vi "Main.vi"(11 "Module Admin":refnum<class "Delacor_lib_QMH_Cloneable Module Admin.lvclass">) -> ()   [LabVIEW 2024, in "RaspberryPiPico.lvlib"]
doc: "This template is based off of the Queued Message Handler design pattern and the Queued Message Handler project template that ships with LabVIEW.\n\nThe main difference is that the queue is private to this module and communication between modules is performed via Broadcast and Request events.\n\nRequest events are wrapped in public API methods and are handled in the Event Handling Loop (EHL) of this VI. Any module can register for Broadcast events sent by this module. The EHL generates messages based on user interface actions.\n\nThe Message Handling Loop (MHL) processes messages generated by the EHL, or by other messages. The messages are string values, so new messages can be added easily to the Message Cases case structure in the MHL. Each message cluster can also provide an optional value for Message Data, which is a variant that can be converted to whatever message-specific data is required.\n_____\nBased on DQMH Dev Tools: Project Template 7.1.0.1503."
uses:
  RaspberryPiPico.lvlib
  <vilib>/Delacor/Delacor QMH/Libraries/Cloneable Module Admin_class/Delacor_lib_QMH_Cloneable Module Admin.lvclass
  C:/Program Files (x86)/National Instruments/LabVIEW 2024/vi.lib/Delacor/Delacor QMH/Libraries/Module Admin_class/Delacor_lib_QMH_Module Admin.lvclass
  Module Data--cluster.ctl
  <vilib>/Delacor/Delacor QMH/Libraries/Cloneable Module Admin_class/Delacor_lib_QMH_Cloneable Module Admin.lvclass/Delacor_lib_QMH_Cloneable Module Admin.ctl
  <vilib>/Delacor/Delacor QMH/Libraries/Message Queue_class/Delacor_lib_QMH_Message Queue.lvclass/Delacor_lib_QMH_Message Queue.ctl
  Stop Argument--cluster.ctl
  <vilib>/Delacor/Delacor QMH/Libraries/Module Admin_class/Delacor_lib_QMH_Module Admin.lvclass/Delacor_lib_QMH_Module Admin.ctl
  Initialize Instrument Argument--cluster.ctl
  Initialize Instrument (Reply Payload)--cluster.ctl
  <instrlib>/HandsOnPi2040/cti-drivers-lv-visa-main/CTI-Visa/Identity.ctl
  <vilib>/Utility/miscctls.llb/LVPointTypeDef.ctl
  <vilib>/Delacor/Delacor QMH/Libraries/Cloneable Module Admin_class/Delacor_lib_QMH_Get Module ID.vi
  <vilib>/Delacor/Delacor QMH/Libraries/Message Queue_class/Delacor_lib_QMH_Enqueue Message (Single).vi
  <vilib>/Delacor/Delacor QMH/Libraries/Module Admin_class/Delacor_lib_QMH_Get External Launch.vi
  <vilib>/Delacor/Delacor QMH/Libraries/Message Queue_class/Delacor_lib_QMH_Message Queue.lvclass
  <instrlib>/HandsOnPi2040/cti-drivers-lv-visa-main/CTI-Visa/CTI-Visa.lvlib
  <instrlib>/HandsOnPi2040/HandsOnPi2040.lvlib
panel:
  out "error out":errorcluster
  out "Status":string
  in  "Simulate EHL Error":bool
  in  "Simulate MHL Error":bool
  # "Other processes communicate with this Module via its Public API (wrappers for its Request Events).\n\nThis Module communicates with other processes via its Broadcast Events.\nAny process that wants to receive these messages can register for this module's Broadcast events."
  # "This template is for the DQMH framework. See the block diagram for more information on how to use this template."
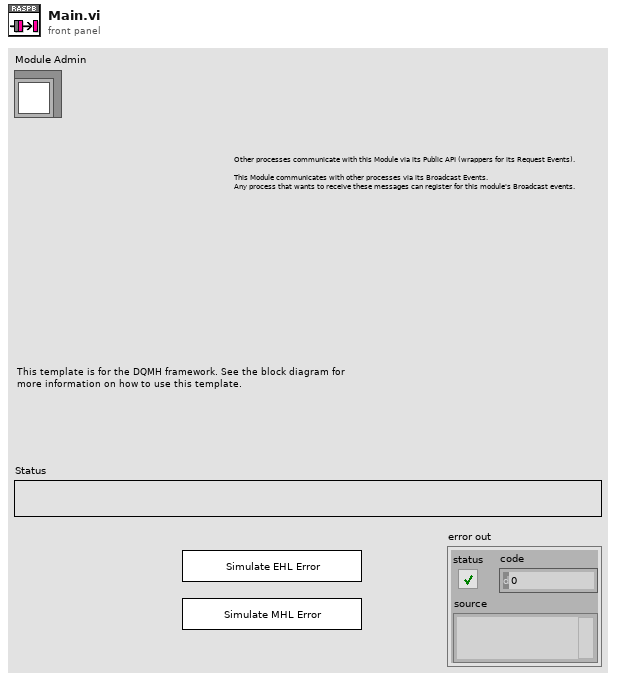
[diagram p1: front panel]
types:
  T1 = typedef "RaspberryPiPico.lvlib/Request Events--cluster.ctl" = cluster{"Stop Module":refnum<user-event>, "Show Panel":refnum<user-event>, "Hide Panel":refnum<user-event>, "Show Diagram":refnum<user-event>, "Get Module Execution Status":refnum<user-event>, "Initialize Instrument":refnum<user-event>, "Local Instance":T2}
  T2 = typedef "RaspberryPiPico.lvlib/Local Instance Request Events--cluster.ctl" = cluster{"Start Continuous Acquisition":refnum<user-event>}
  T3 = typedef "RaspberryPiPico.lvlib/Module Data--cluster.ctl" = cluster{"Status":string, "VISA resource name":refnum<visa-resource-name>}
  T4 = enum32{"invalid lock state", "Not Locked", "Locked (No Password)", "Password-protected"}
  T5 = typedef "RaspberryPiPico.lvlib/Stop Argument--cluster.ctl" = cluster{"Module ID":i32, "Origin":string, "Exit via Stop Module Req?":bool, "Wait for Module to stop?":bool}
  T6 = typedef "RaspberryPiPico.lvlib/Initialize Instrument Argument--cluster.ctl" = cluster{"Module ID":i32, "VISA resource name":refnum<visa-resource-name>, "Wait Notifier":refnum<notifier>, "wait for reply":bool}
  T7 = typedef "LVPointTypeDef.ctl" = cluster{"Horizontal":i16, "Vertical":i16}
  T8 = enum32{"Invalid", "Standard", "Closed", "Hidden", "Minimized", "Maximized"}
  T9 = typedef "RaspberryPiPico.lvlib/Initialize Instrument (Reply Payload)--cluster.ctl" = cluster{"Module ID":i32, "Identity":T10, "error":errorcluster}
  T10 = typedef "CTI-Visa.lvlib/Identity.ctl" = cluster{"Vendor":string, "Model":string, "Serial":string, "Version":string}
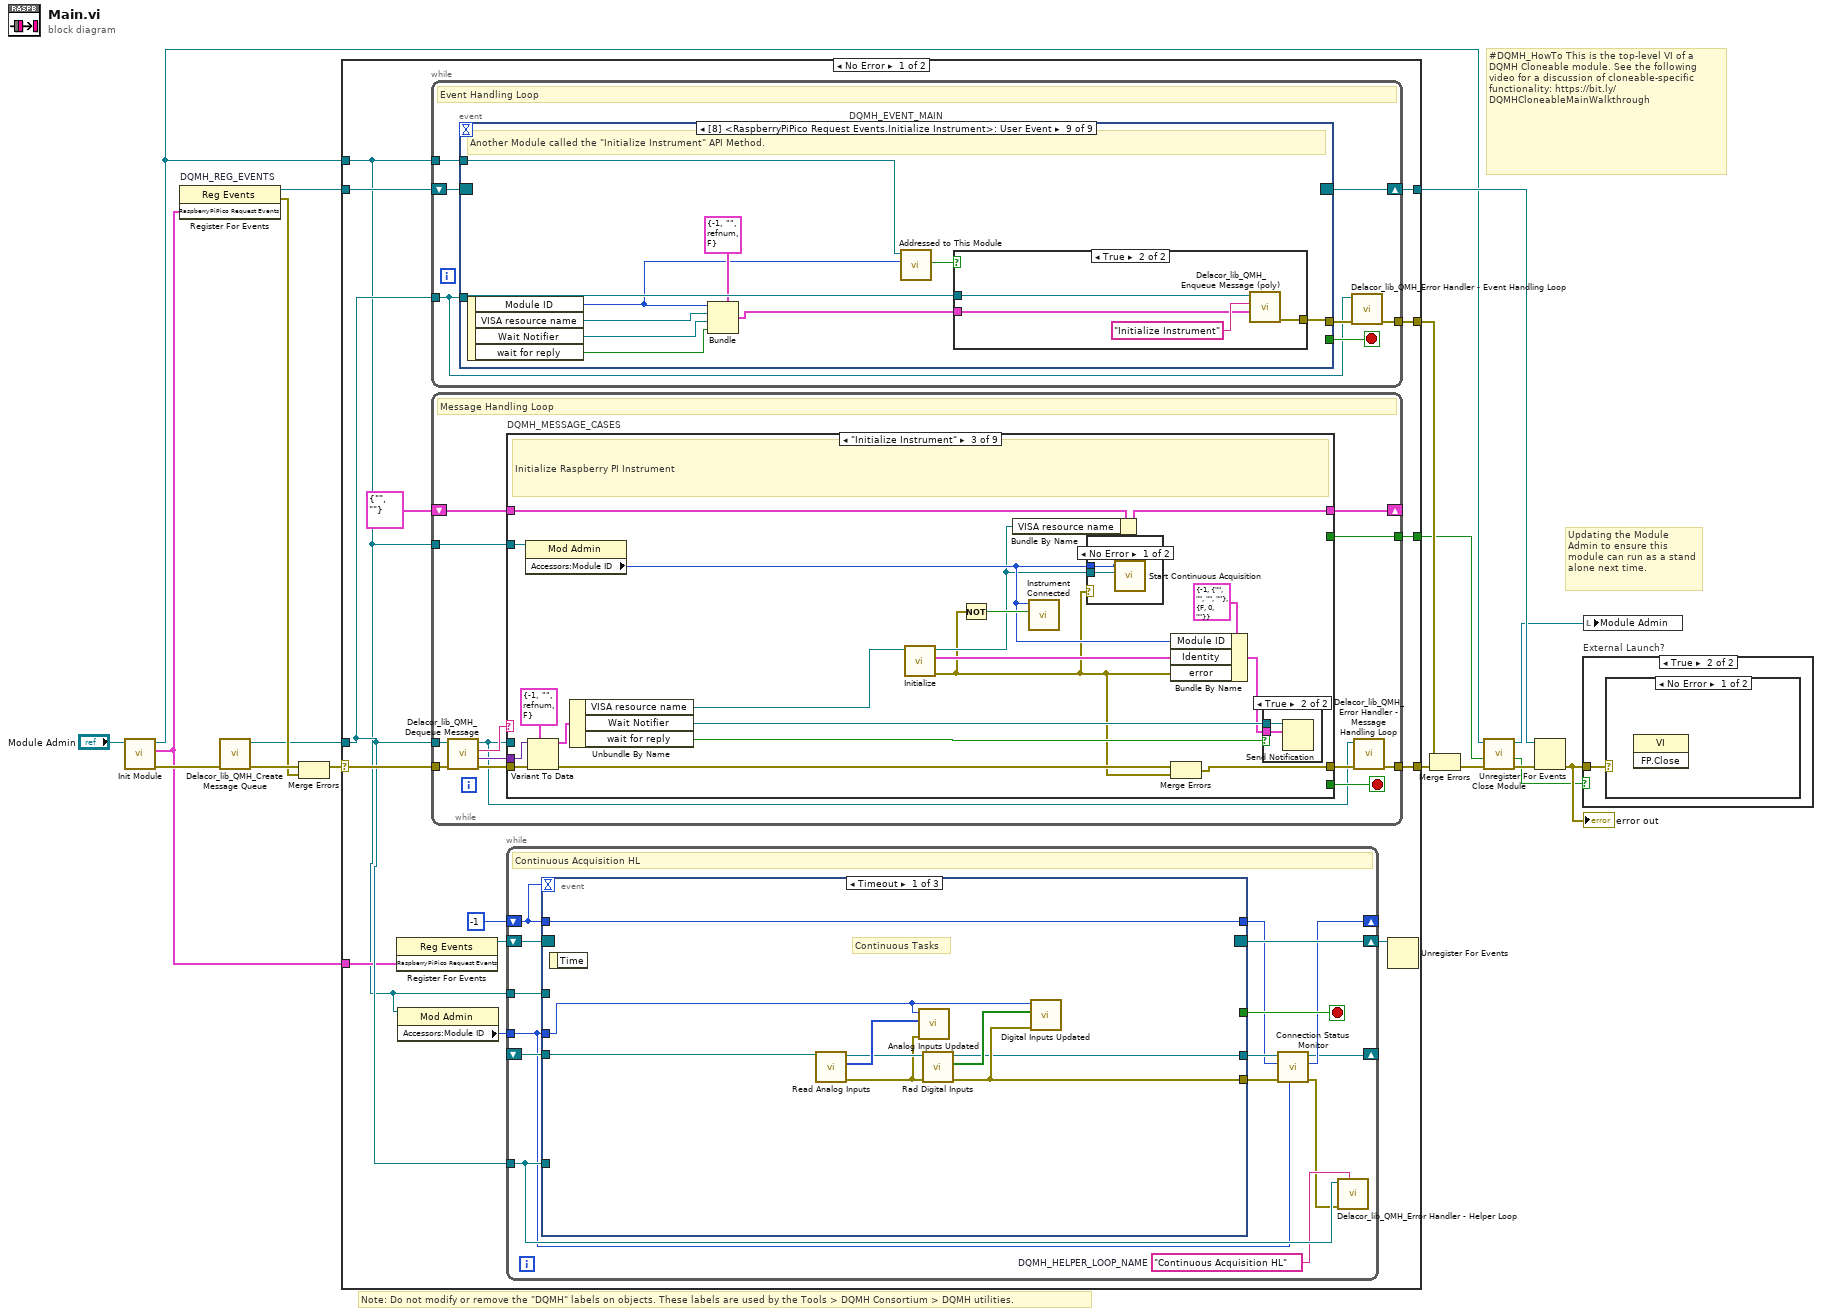
[diagram p0: block diagram]
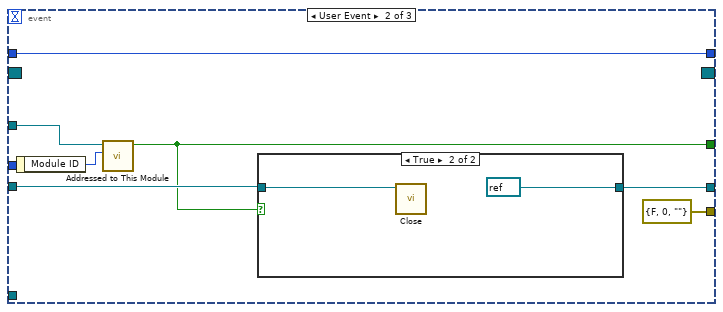
[diagram p2: hidden frame]
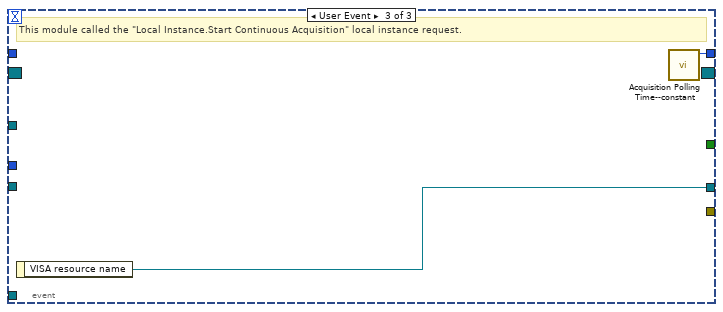
[diagram p4: hidden frame]
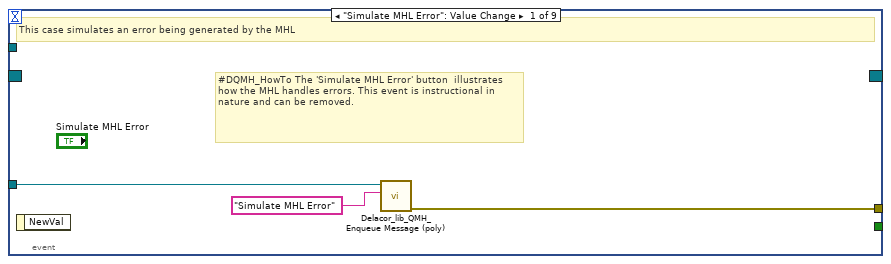
[diagram p5: hidden frame]
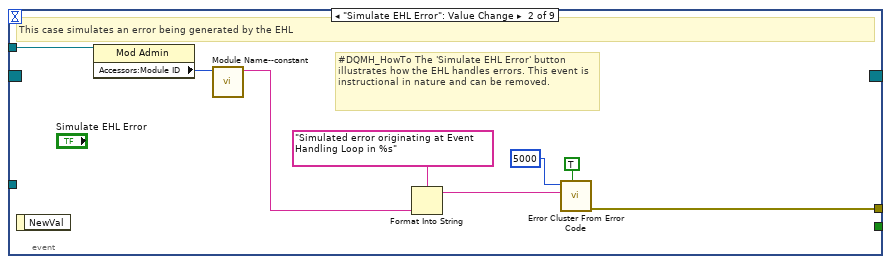
[diagram p6: hidden frame]
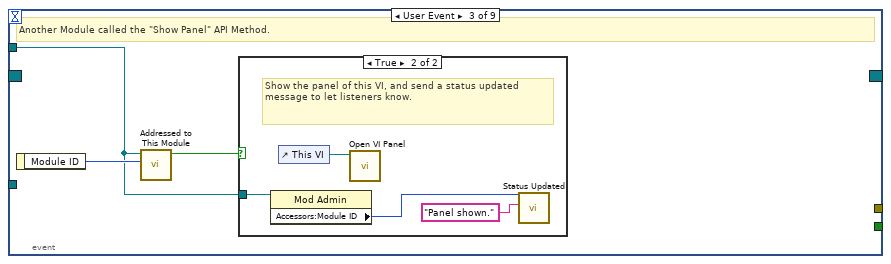
[diagram p7: hidden frame]
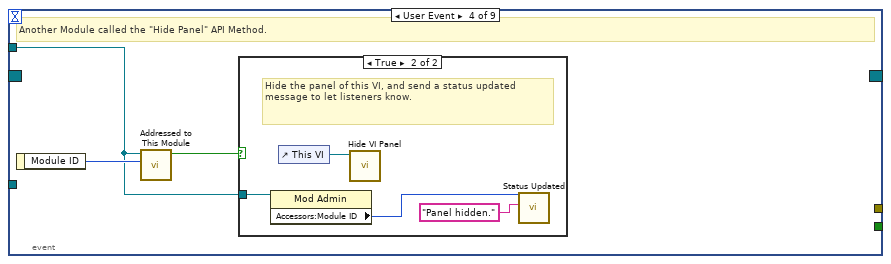
[diagram p9: hidden frame]
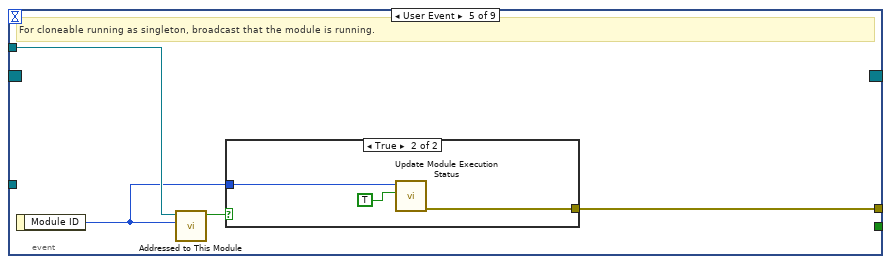
[diagram p11: hidden frame]
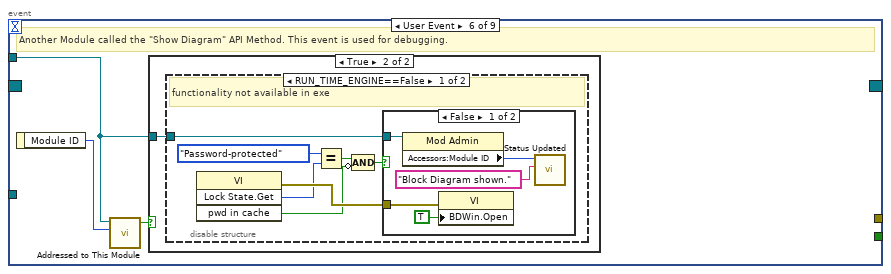
[diagram p13: hidden frame]
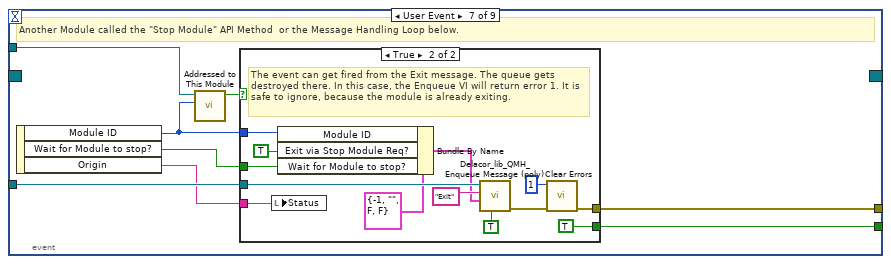
[diagram p17: hidden frame]
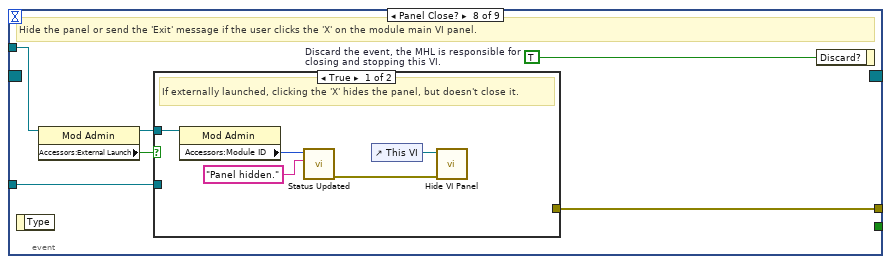
[diagram p19: hidden frame]
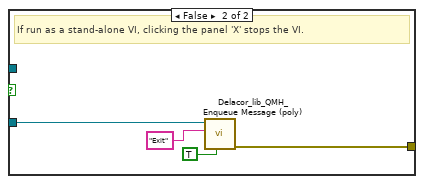
[diagram p20: hidden frame]
diagram:
  # "#DQMH_HowTo This is the top-level VI of a DQMH Cloneable module. See the following video for a discussion of cloneable-specific functionality: https://bit.ly/DQMHCloneableMainWalkthrough"
  # "Note: Do not modify or remove the \"DQMH\" labels on objects. These labels are used by the Tools > DQMH Consortium > DQMH utilities."
  # "Updating the Module Admin to ensure this module can run as a stand alone next time."
  n1 = call "Init Module.vi"("Cloneable Module Admin in"="Module Admin") -> ("error out"=w15:errorcluster, "RaspberryPiPico Request Events"=w1:T1, "Cloneable Module Admin out"=w5:refnum<class "Delacor_lib_QMH_Cloneable Module Admin.lvclass">)  [unwired: 8 in]
  n2 = register-events "DQMH_REG_EVENTS"(w1) -> (reference out=w8:refnum<event-registration>, error out=w10:errorcluster)  [unwired: 2 in]
  n3 = call <vilib>:"Delacor_lib_QMH_Create Message Queue.vi"("error in"=w15) -> ("error out"=w12:errorcluster, "Message Queue"=w7:refnum<class "Delacor_lib_QMH_Message Queue.lvclass">)  [unwired: 9 in]
  n4 = Merge Errors(w12, w10) -> (w11:errorcluster)
  n5 = case shown="No Error" w11 {
    selector: w11 -> [w30 w307]
    tunnel: [w32 w306] -> w16
    tunnel: [w29 w305] -> w9
    tunnel: w8 -> [w27 w305]
    tunnel: w7 -> [w26 w298]
    tunnel: [w31 _] -> w17
    tunnel: w5 -> [w20 w301]
    tunnel: [w25 _] -> w3
    tunnel: w1 -> [w24 _]
    frame No Error {
      n6 = register-events ("DQMH_HELPER_REGFOREVENTS")(w24) -> (reference out=w22:refnum<event-registration>)  [unwired: 2 in, 1 out]
      n7 = property class="Mod Admin"(reference=w20) -> ("Accessors:Module ID"=w19:i32)  [unwired: 1 in, 2 out]
      n8 = while {
        tunnel: w26 -> [w70]
        shift-right: [w73] -> w29
        shift-left: w27 -> [w74]
        tunnel: [w75] -> w31
        tunnel: w20 -> [w71]
        stop <- w72 stop-if-true
        # "Event Handling Loop"
        n9 = event "DQMH_EVENT_MAIN" shown="[8] <RaspberryPiPico Request Events.Initialize Instrument>: User Event" {
          selector: w74 -> [_ _ _ _ _ _ _ _ _]
          dyn-events: [_ _ _ _ _ _ _ _ _] -> w73
          timeout: _ -> [_ _ _ _ _ _ _ _ _]
          tunnel: [_ _ _ _ _ _ w128 _ _] -> w72
          tunnel: w70 -> [w78 _ _ _ _ _ w131 w148 w169]
          tunnel: [w79 w87 _ _ w105 _ w132 w151 w170] -> w76
          tunnel: w71 -> [_ w86 w88 w95 w103 w109 w130 w149 w167]
          event "Simulate MHL Error": Value Change {
            # "#DQMH_HowTo The 'Simulate MHL Error' button  illustrates how the MHL handles errors. This event is instructional in nature and can be removed."
            # "This case simulates an error being generated by the MHL"
            n10 = event-data() -> ()  [unwired: 1 in, 1 out]
            n11 = call-poly <vilib>:"Delacor_lib_QMH_Enqueue Message (poly).vi"("Message"="Simulate MHL Error", "Message Queue in"=w78) -> ("error out"=w79:errorcluster)  [unwired: 8 in, 1 out]
          }
          event "Simulate EHL Error": Value Change {
            # "#DQMH_HowTo The 'Simulate EHL Error' button  illustrates how the EHL handles errors. This event is instructional in nature and can be removed."
            # "This case simulates an error being generated by the EHL"
            n12 = event-data() -> ()  [unwired: 1 in, 1 out]
            n13 = property on="Property Node" class="Mod Admin"(reference=w86) -> ("Accessors:Module ID"=w85:i32)  [unwired: 1 in, 2 out]
            n14 = call "Module Name--constant.vi"("Module ID"=w85) -> ("Module Name"=w80:string)  [unwired: 10 in]
            n15 = Format Into String(format string="Simulated error originating at Event Handling Loop in %s", w80) -> (resulting string=w83:string)  [unwired: 2 in, 1 out]
            n16 = call <vilib>:"Error Cluster From Error Code.vi"("show call chain? (False)"=TRUE, "error message (\"\")"=w83, "error code (0)"=5000) -> ("error out"=w87:errorcluster)  [unwired: 6 in]
          }
          event User Event {
            # "Another Module called the \"Show Panel\" API Method."
            n17 = event-data() -> ("Module ID"=w89:i32)  [unwired: 1 in]
            n18 = call "Addressed to This Module.vi"("Module ID from Argument"=w89, "Module Admin"=w88) -> ("Addressed to this instance?"=w90:bool)  [unwired: 8 in, 1 out]
            n19 = case shown="True" w90 {
              tunnel: w88 -> [_ w92]
              frame False {
              }
              frame True {
                # "Show the panel of this VI, and send a status updated message to let listeners know."
                n20 = property on="Property Node" class="Mod Admin"(reference=w92) -> ("Accessors:Module ID"=w91:i32)  [unwired: 1 in, 2 out]
                n21 = control-ref of="This VI"() -> (w94:refnum<vi>)
                n22 = call "Open VI Panel.vi"("VI"=w94) -> ()  [unwired: 10 in, 1 out]
                n23 = call "Status Updated.vi"("Status"="Panel shown." ("format string"), "Module ID"=w91) -> ()  [unwired: 9 in, 1 out]
              }
            }
          }
          event User Event {
            # "Another Module called the \"Hide Panel\" API Method."
            n24 = event-data() -> ("Module ID"=w96:i32)  [unwired: 1 in]
            n25 = call "Addressed to This Module.vi"("Module ID from Argument"=w96, "Module Admin"=w95) -> ("Addressed to this instance?"=w97:bool)  [unwired: 8 in, 1 out]
            n26 = case shown="True" w97 {
              tunnel: w95 -> [_ w99]
              frame False {
              }
              frame True {
                # "Hide the panel of this VI, and send a status updated message to let listeners know."
                n27 = property on="Property Node" class="Mod Admin"(reference=w99) -> ("Accessors:Module ID"=w98:i32)  [unwired: 1 in, 2 out]
                n28 = control-ref of="This VI"() -> (w101:refnum<vi>)
                n29 = call "Hide VI Panel.vi"("VI"=w101) -> ()  [unwired: 10 in, 1 out]
                n30 = call "Status Updated.vi"("Status"="Panel hidden." ("format string"), "Module ID"=w98) -> ()  [unwired: 9 in, 1 out]
              }
            }
          }
          event User Event {
            # "For cloneable running as singleton, broadcast that the module is running."
            n31 = event-data() -> ("Module ID"=w102:i32)  [unwired: 1 in]
            n32 = call "Addressed to This Module.vi"("Module ID from Argument"=w102, "Module Admin"=w103) -> ("Addressed to this instance?"=w104:bool)  [unwired: 8 in, 1 out]
            n33 = case shown="True" w104 {
              tunnel: [_ w108] -> w105
              tunnel: w102 -> [_ w107]
              frame False {
              }
              frame True {
                n34 = call "Update Module Execution Status.vi"("Running?"=TRUE, "Module ID"=w107) -> ("error out"=w108:errorcluster)  [unwired: 9 in]
              }
            }
          }
          event User Event {
            # "Another Module called the \"Show Diagram\" API Method. This event is used for debugging."
            n35 = event-data() -> ("Module ID"=w110:i32)  [unwired: 1 in]
            n36 = call "Addressed to This Module.vi"("Module ID from Argument"=w110, "Module Admin"=w109) -> ("Addressed to this instance?"=w111:bool)  [unwired: 8 in, 1 out]
            n37 = case shown="True" w111 {
              tunnel: w109 -> [_ w112]
              frame False {
              }
              frame True {
                n38 = disable-structure shown="RUN_TIME_ENGINE==False" {
                  disable-tunnel: w112 -> [w113 _]
                  frame condition #0 (active) {
                    # "functionality not available in exe"
                    n39 = invoke on="Invoke Node" class="VI" method="Lock State.Get"() -> (error out=w119:errorcluster, "Get Lock State"=w118:T4, "pwd in cache"=w115:bool)  [unwired: 4 in, 1 out]
                    n40 = Equal?(x=T4."Password-protected", y=w118) -> (x = y?=w116:bool)
                    n41 = Compound Arithmetic op=AND(w116, invert w115) -> (w114:bool)
                    n42 = case shown="False" w114 {
                      tunnel: w119 -> [w124 _]
                      tunnel: w113 -> [w121 _]
                      frame False {
                        n43 = property on="Property Node" class="Mod Admin"(reference=w121) -> ("Accessors:Module ID"=w120:i32)  [unwired: 1 in, 2 out]
                        n44 = property on="Property Node" class="VI"(error in=w124, "BDWin.Open"=TRUE ("Block Diagram Window:Open")) -> ()  [unwired: 1 in, 2 out]
                        n45 = call "Status Updated.vi"("Status"="Block Diagram shown." ("format string"), "Module ID"=w120) -> ()  [unwired: 9 in, 1 out]
                      }
                      frame True {
                        # "Password-protected VI, and the password is not in the cache. Do not show the diagram."
                      }
                    }
                  }
                  frame condition #1 {
                  }
                }
              }
            }
          }
          event User Event {
            # "Another Module called the \"Stop Module\" API Method  or the Message Handling Loop below."
            n46 = event-data() -> ("Module ID"=w126:i32, "Wait for Module to stop?"=w127:bool, "Origin"=w125:string)  [unwired: 1 in]
            n47 = call "Addressed to This Module.vi"("Module ID from Argument"=w126, "Module Admin"=w130) -> ("Addressed to this instance?"=w129:bool)  [unwired: 8 in, 1 out]
            n48 = case shown="True" w129 {
              tunnel: [_ w144] -> w132
              tunnel: w131 -> [_ w140]
              tunnel: [_ TRUE] -> w128
              tunnel: w127 -> [_ w135]
              tunnel: w126 -> [_ w137]
              tunnel: w125 -> [_ w133]
              frame False {
              }
              frame True {
                # "The event can get fired from the Exit message. The queue gets destroyed there. In this case, the Enqueue VI will return error 1. It is safe to ignore, because the module is already exiting."
                n49 = local write "Status"(w133) -> ()
                n50 = Bundle By Name(cluster=T5 {"Module ID"=-1, "Origin"="", "Exit via Stop Module Req?"=FALSE, "Wait for Module to stop?"=FALSE} ("Stop Argument"), "Module ID"=w137, "Exit via Stop Module Req?"=TRUE, "Wait for Module to stop?"=w135) -> (w134:T5)
                n51 = call-poly <vilib>:"Delacor_lib_QMH_Enqueue Message (poly).vi"("Priority Message? (F)"=TRUE, "Message Data"=w134, "Message"="Exit", "Message Queue in"=w140) -> ("error out"=w145:errorcluster)  [unwired: 6 in, 1 out]
                n52 = call <vilib>:"Clear Errors.vi"("error in (no error)"=w145, "specific error code to clear (0: all)"=1) -> ("error out"=w144:errorcluster)  [unwired: 4 in, 1 out]
              }
            }
          }
          event Panel Close? {
            w150 = TRUE  # Discard the event, the MHL is responsible for closing and stopping this VI.
            # "Hide the panel or send the 'Exit' message if the user clicks the 'X' on the module main VI panel."
            n53 = event-data() -> ()  [unwired: 1 in, 1 out]
            n54 = property on="Property Node" class="Mod Admin"(reference=w149) -> (reference out=w146:refnum<class "Delacor_lib_QMH_Cloneable Module Admin.lvclass">, "Accessors:External Launch"=w147:bool)  [unwired: 1 in, 1 out]
            n55 = case shown="True" w147 {
              tunnel: w148 -> [_ w159]
              tunnel: [_ w160] -> w151
              tunnel: w146 -> [w153 _]
              frame True {
                # "If externally launched, clicking the 'X' hides the panel, but doesn't close it."
                n56 = property on="Property Node" class="Mod Admin"(reference=w153) -> ("Accessors:Module ID"=w152:i32)  [unwired: 1 in, 2 out]
                n57 = call "Status Updated.vi"("Status"="Panel hidden." ("format string"), "Module ID"=w152) -> ("error out"=w156:errorcluster)  [unwired: 9 in]
                n58 = control-ref of="This VI"() -> (w155:refnum<vi>)
                n59 = call "Hide VI Panel.vi"("error in"=w156, "VI"=w155) -> ()  [unwired: 9 in, 1 out]
              }
              frame False {
                # "If run as a stand-alone VI, clicking the panel 'X' stops the VI."
                n60 = call-poly <vilib>:"Delacor_lib_QMH_Enqueue Message (poly).vi"("Priority Message? (F)"=TRUE, "Message"="Exit", "Message Queue in"=w159) -> ("error out"=w160:errorcluster)  [unwired: 7 in, 1 out]
              }
            }
            n61 = event-data ("Event Filter Node")("Discard?"=w150) -> ()  [unwired: 1 in, 1 out]
          }
          event User Event {
            # "Another Module called the \"Initialize Instrument\" API Method."
            n62 = event-data() -> ("Module ID"=w164:i32, "VISA resource name"=w163:refnum<visa-resource-name>, "Wait Notifier"=w162:refnum<notifier>, "wait for reply"=w161:bool)  [unwired: 1 in]
            n63 = Bundle(cluster=T6 {"Module ID"=-1, "VISA resource name"="", "Wait Notifier"=refnum, "wait for reply"=FALSE} ("Initialize Instrument Argument"), "Module ID"=w164, "VISA resource name"=w163, "Wait Notifier"=w162, "wait for reply"=w161) -> (w165:T6)
            n64 = call "Addressed to This Module.vi"("Module ID from Argument"=w164, "Module Admin"=w167) -> ("Addressed to this instance?"=w168:bool)  [unwired: 8 in, 1 out]
            n65 = case shown="True" w168 {
              tunnel: w169 -> [_ w173]
              tunnel: w165 -> [_ w171]
              tunnel: [_ w174] -> w170
              frame False {
              }
              frame True {
                n66 = call-poly <vilib>:"Delacor_lib_QMH_Enqueue Message (poly).vi"("Message Data"=w171, "Message"="Initialize Instrument", "Message Queue in"=w173) -> ("error out"=w174:errorcluster)  [unwired: 7 in, 1 out]
              }
            }
          }
        }
        n67 = call-dynamic "Delacor_lib_QMH_Error Handler - Event Handling Loop.vi"("error in"=w76, "Message Queue in"=w70) -> ("dup error in"=w75:errorcluster)  [unwired: 8 in, 1 out]
      }
      n68 = while {
        tunnel: w26 -> [w175]
        shift-right: [w182] -> _
        shift-left: T3 {"Status"="", "VISA resource name"=""} ("Data Cluster") -> [w183]
        tunnel: w30 -> [w186]
        tunnel: [w184] -> w32
        tunnel: w20 -> [w177]
        tunnel: [w176] -> w25
        stop <- w181 stop-if-true
        # "Message Handling Loop"
        n69 = call-dynamic "Delacor_lib_QMH_Dequeue Message.vi"("error in"=w186, "Message Queue in"=w175) -> ("error out"=w185:errorcluster, "Message Data"=w179:variant, "Message"=w180:string, "Message Queue out"=w178:refnum<class "Delacor_lib_QMH_Message Queue.lvclass">)  [unwired: 6 in]
        n70 = case "DQMH_MESSAGE_CASES" shown="\"Initialize Instrument\"" w180 {
          selector: w180 -> [_ _ _ _ _ _ _ _ w287]
          tunnel: w178 -> [_ _ _ _ _ w240 _ w279 _]
          tunnel: w185 -> [w206 w210 w229 w236 w238 w250 w267 w285 w296]
          tunnel: [w204 w210 w227 w235 w238 w246 w266 w280 w297] -> w187
          tunnel: w183 -> [w197 w209 w226 w234 w237 w244 w264 w269 w294]
          tunnel: [w196 w209 w216 w234 w237 w244 w264 w269 w294] -> w182
          tunnel: [_ _ _ _ _ _ _ w278 _] -> w181
          tunnel: w179 -> [_ _ w225 _ _ w243 _ w276 _]
          tunnel: w177 -> [w192 _ w218 _ _ w242 w262 w271 w293]
          tunnel: [_ _ _ _ _ _ _ w274 _] -> w176
          frame "Initialize" {
            w189 = "Initial Message" ("Initial Message")
            # "#DQMH_CodeNeeded - Initialize the appearance of the front panel."
            # "#DQMH_CodeNeeded - Initialize your state data here."
            # "Initialize - Any operation that needs to be done before the module can receive messages. Synchronize Caller Events.vi will inform Start Module.vi that the module has launched and is ready to receive messages. Module Did Init.vi will broadcast that the module initialized."
            n71 = call "Synchronize Caller Events.vi"("error in"=w206, "Module Admin"=w192) -> ("error out"=w205:errorcluster, "Module Admin out"=w191:refnum<class "Delacor_lib_QMH_Cloneable Module Admin.lvclass">)  [unwired: 8 in]
            n72 = property on="Property Node" class="Mod Admin"(reference=w191) -> ("Accessors:Module ID"=w188:i32, "Accessors:External Launch"=w193:bool)  [unwired: 1 in, 2 out]
            n73 = call "Module Name--constant.vi"("Module ID"=w188) -> ("Module Name"=w201:string)  [unwired: 10 in]
            n74 = property on="Property Node" class="VI"("Front Panel.Title"=w201) -> (reference out=w203:refnum<vi>, error out=w208:errorcluster)  [unwired: 2 in]
            n75 = Select(t=T8."Hidden" ("State"), s=w193, f=T8."Standard" ("State")) -> (s? t:f=w198:T8)
            n76 = invoke on="Invoke Node" class="VI" method="FP.Open"(reference=w203, error in=w208, "State"=w198) -> (reference out=w202:refnum<vi>, error out=w207:errorcluster)  [unwired: 2 in, 3 out]
            n77 = Bundle By Name(cluster=w197, "Status"=w189) -> (w196:T3)
            n78 = invoke on="Invoke Node" class="VI" method="FP.Center"(reference=w202, error in=w207) -> ()  [unwired: 1 in, 3 out]
            n79 = property on="Pane" class="Pane"("Origin"=T7 {"Horizontal"=0, "Vertical"=0}) -> ()  [unwired: 2 in, 2 out]
            n80 = call "Module Name--constant.vi"("Module ID"=w188) -> ("Module Name"=w194:string)  [unwired: 10 in]
            n81 = call "Module Did Init.vi"("error in"=w205, "Initialized?"=TRUE, "Origin"=w194, "Module ID"=w188) -> ("error out"=w204:errorcluster)  [unwired: 7 in]
            "Status" <- w189
          }
          frame "---Module Specific---" {
            # "Separator -- The following cases handle messages specific to this Module."
          }
          frame "Initialize Instrument" {
            # "Initialize Raspberry PI Instrument"
            n82 = property class="Mod Admin"(reference=w218) -> ("Accessors:Module ID"=w213:i32)  [unwired: 1 in, 2 out]
            n83 = Variant To Data(error in=w229, type=T6 {"Module ID"=-1, "VISA resource name"="", "Wait Notifier"=refnum, "wait for reply"=FALSE} ("Initialize Instrument Argument"), Variant=w225) -> (data=w223:T6, error out=w228:errorcluster)
            n84 = Unbundle By Name(w223) -> ("VISA resource name"=w215:refnum<visa-resource-name>, "Wait Notifier"=w222:refnum<notifier>, "wait for reply"=w221:bool)
            n85 = call <instrlib>:"Initialize.vi"("VISA resource name"=w215) -> ("error out"=w211:errorcluster, "Identity"=w217:T10, "VISA resource name out"=w212:refnum<visa-resource-name>)  [unwired: 8 in]
            n86 = Not(x=w211) -> (.not. x?=w214:bool)
            n87 = Bundle By Name(cluster=w226, "VISA resource name"=w212) -> (w216:T3)
            n88 = call "Instrument Connected.vi"("Instrument Connection Status"=w214, "Module ID"=w213) -> ()  [unwired: 9 in, 1 out]
            n89 = case shown="No Error" w211 {
              tunnel: w213 -> [w231 _]
              tunnel: w212 -> [w230 _]
              frame No Error {
                n90 = call "Start Continuous Acquisition.vi"("VISA resource name"=w230, "Module ID"=w231) -> ()  [unwired: 9 in, 1 out]
              }
              frame Error {
              }
            }
            n91 = Bundle By Name(cluster=T9 {"Module ID"=-1, "Identity"={"Vendor"="", "Model"="", "Serial"="", "Version"=""}, "error"={"status"=FALSE, "code"=0, "source"=""}} ("Initialize Instrument (Reply Payload)"), "Module ID"=w213, "Identity"=w217, "error"=w211) -> (w220:T9)
            n92 = Merge Errors(w228, w211) -> (w227:errorcluster)
            n93 = case "DQMH_FIRE_NOTIFIER" shown="True" w221 {
              tunnel: w222 -> [_ w233]
              tunnel: w220 -> [_ w232]
              frame False {
              }
              frame True {
                n94 = Send Notification(notification=w232, notifier=w233) -> ()  [unwired: 1 in, 2 out]
              }
            }
          }
          frame "---Copy This Frame---" {
            # "Duplicate this frame when creating new messages.  Change this comment in the duplicated frame to describe this message."
            n95 = Merge Errors(w236) -> (w235:errorcluster)
          }
          frame "---Exit and Error Handling---" {
            # "Separator - the following cases handle errors and exit messages."
          }
          frame "Error" {
            # "#DQMH_CodeRecommended - If the module is running in standalone mode (External Launch = FALSE), this code will pop up an error dialog and call the 'Exit' message if an error occurs. Add more fine-grained error management here."
            # "Error - Check the error message data and respond accordingly. This message is sent by the \"Error Handler\" VIs at the end of each loop in this application."
            n96 = property on="Property Node" class="Mod Admin"(reference=w242) -> ("Accessors:External Launch"=w241:bool, "Accessors:Module ID"=w239:i32)  [unwired: 1 in, 2 out]
            n97 = Variant To Data(error in=w250, type=errorcluster {"status"=FALSE, "code"=0, "source"=""} ("error constant"), Variant=w243) -> (data=w245:errorcluster, error out=w248:errorcluster)
            n98 = local write "error out"(w245) -> ()
            n99 = call "Error Reported.vi"("Error"=w245, "Module ID"=w239) -> ()  [unwired: 9 in, 1 out]
            n100 = case shown="False" w241 {
              tunnel: [w255 _] -> w247
              tunnel: w240 -> [w253 _]
              tunnel: w245 -> [w254 _]
              frame False {
                n101 = disable-structure shown="Default" {
                  disable-tunnel: w254 -> [w256 _]
                  frame condition #0 (active) {
                    # "If the module is running standalone, then pop up an error dialog and call the \"Exit\" message."
                    n102 = call <vilib>:"Simple Error Handler.vi"("error in (no error)"=w256) -> ()  [unwired: 4 in, 5 out]
                  }
                  frame condition #1 {
                    # "To prevent the Simple Error Handler VI from being loaded (e.g. when deploying to a Real-Time target), add the Conditional Disable Symbol \"DQMH_Disable_SEH\" to your project and set it to TRUE."
                  }
                }
                n103 = call-poly <vilib>:"Delacor_lib_QMH_Enqueue Message (poly).vi"("Priority Message? (F)"=TRUE, "Message"="Exit", "Message Queue in"=w253) -> ("error out"=w255:errorcluster)  [unwired: 7 in, 1 out]
              }
              frame True {
                # "If the module was launched externally, calling the Error Reported broadcast VI is the only action performed by the \"Error\" message. The module's caller can then process the error appropriately."
              }
            }
            n104 = Merge Errors(w248, w247) -> (w246:errorcluster)
          }
          frame "Simulate MHL Error" {
            # "#DQMH_HowTo The 'Simulate MHL Error' button  illustrates how the MHL handles errors. This event is instructional in nature and can be removed."
            # "Simulate an error occurring at the MHL"
            n105 = property on="Property Node" class="Mod Admin"(reference=w262) -> ("Accessors:Module ID"=w263:i32)  [unwired: 1 in, 2 out]
            n106 = call "Module Name--constant.vi"("Module ID"=w263) -> ("Module Name"=w258:string)  [unwired: 10 in]
            n107 = Format Into String(format string="Simulated error originating at Message Handling Loop in %s", w258) -> (resulting string=w259:string)  [unwired: 2 in, 1 out]
            n108 = call <vilib>:"Error Cluster From Error Code.vi"("show call chain? (False)"=TRUE, "error message (\"\")"=w259, "error code (0)"=5001) -> ("error out"=w265:errorcluster)  [unwired: 6 in]
            n109 = Merge Errors(w267, w265) -> (w266:errorcluster)
          }
          frame "Exit" {
            w277 = 91  # 91: not all Exit messages will have an argument
            w278 = TRUE  # Stop the VI
            # "Release the message queue reference"
            # "#DQMH_CodeNeeded - Add any required cleanup code here."
            # "Exit - Exit the application."
            n110 = Variant To Data(error in=w285, type=T5 {"Module ID"=-1, "Origin"="", "Exit via Stop Module Req?"=FALSE, "Wait for Module to stop?"=FALSE} ("Stop Argument"), Variant=w276) -> (data=w273:T5, error out=w281:errorcluster)
            n111 = call <vilib>:"Clear Errors.vi"("error in (no error)"=w281, "specific error code to clear (0: all)"=w277) -> ("error out"=w284:errorcluster)  [unwired: 4 in, 1 out]
            n112 = property on="Property Node" class="Mod Admin"(reference=w271) -> ("Accessors:Module ID"=w270:i32)  [unwired: 1 in, 2 out]
            n113 = control-ref of="This VI"() -> (w272:refnum<vi>)
            n114 = call-dynamic "Delacor_lib_QMH_Release Message Queue.vi"("error in"=w284, "Message Queue"=w279) -> ("error out"=w283:errorcluster)  [unwired: 9 in]
            n115 = call "Handle Exit.vi"("Stop Argument"=w273, "Module Admin in"=w271, "VI reference"=w272) -> ("error out"=w282:errorcluster, "Wait for Stop?"=w274:bool)  [unwired: 7 in]
            n116 = Merge Errors(w283, w282) -> (w280:errorcluster)
            n117 = call "Error Reported.vi"("Error"=w280, "Module ID"=w270) -> ()  [unwired: 9 in, 1 out]
            n118 = Unbundle By Name(w269) -> ("VISA resource name"=w268:refnum<visa-resource-name>)
            n119 = call <instrlib>:"Close.vi"("VISA resource name"=w268) -> ()  [unwired: 10 in, 1 out]
          }
          frame Default {
            # "'Default' case only runs if there is a message that isn't defined in any of the other cases.  Output a programming error."
            n120 = property on="Property Node" class="Mod Admin"(reference=w293) -> ("Accessors:Module ID"=w292:i32)  [unwired: 1 in, 2 out]
            n121 = call "Module Name--constant.vi"("Module ID"=w292) -> ("Module Name"=w286:string)  [unwired: 10 in]
            n122 = Format Into String(format string="The invalid message string \"%s\" was received in the Message Handling Loop for module \"%s\".", w287, w286) -> (resulting string=w289:string)  [unwired: 2 in, 1 out]
            n123 = call <vilib>:"Error Cluster From Error Code.vi"("show call chain? (False)"=TRUE, "error message (\"\")"=w289, "error code (0)"=1) -> ("error out"=w295:errorcluster)  [unwired: 6 in]
            n124 = Merge Errors(w296, w295) -> (w297:errorcluster)
          }
        }
        n125 = call-dynamic "Delacor_lib_QMH_Error Handler - Message Handling Loop.vi"("error in"=w187, "Message Queue in"=w178) -> ("dup error in"=w184:errorcluster)  [unwired: 8 in, 1 out]
      }
      n126 = while "DQMH_HELPER_LOOP" {
        shift-right: [w38] -> _
        shift-left: -1 -> [w47]
        shift-right: [w45] -> w23
        shift-left: w22 -> [w46]
        tunnel: w26 -> [w43]
        tunnel: w20 -> [w41]
        shift-right: [w37] -> _
        shift-left: _ -> [w40]
        tunnel: w19 -> [w33]
        stop <- w44 stop-if-true
        w42 = "Continuous Acquisition HL"  # DQMH_HELPER_LOOP_NAME
        # "Continuous Acquisition HL"
        n127 = event "DQMH_HELPER_EVENT_STRUCTURE" shown="[0] Timeout" {
          selector: w46 -> [_ _ _]
          dyn-events: [_ _ _] -> w45
          timeout: w47 -> [_ _ _]
          tunnel: w47 -> [w51 w64 _]
          tunnel: [w51 w64 w68] -> w34
          tunnel: [_ w59 _] -> w44
          tunnel: w43 -> [_ _ _]
          tunnel: w41 -> [w49 w63 _]
          tunnel: [w50 w60 w69] -> w36
          tunnel: w40 -> [w57 w61 _]
          tunnel: [w52 errorcluster {"status"=FALSE, "code"=0, "source"=""} ("error constant") _] -> w39
          tunnel: [w49 _ _] -> _
          tunnel: w33 -> [w48 _ _]
          event Timeout {
            # "Continuous Tasks"
            n128 = event-data() -> ()  [unwired: 1 in, 1 out]
            n129 = call "Read Analog Inputs.vi"("VISA Refnum in"=w57) -> ("error out"=w53:errorcluster, "Analog Inputs"=w56:u16[], "VISA Refnum out"=w55:refnum<visa-resource-name>)  [unwired: 8 in]
            n130 = call "Analog Inputs Updated.vi"("error in"=w53, "Analog Inputs"=w56, "Module ID"=w48) -> ()  [unwired: 8 in, 1 out]
            n131 = call "Rad Digital Inputs.vi"("error In"=w53, "VISA Refnum in"=w55) -> ("error out"=w52:errorcluster, "Digital Inputs"=w54:bool[], "VISA Refnum out"=w50:refnum<visa-resource-name>)  [unwired: 7 in]
            n132 = call "Digital Inputs Updated.vi"("error in"=w52, "Digital Inputs"=w54, "Module ID"=w48) -> ()  [unwired: 8 in, 1 out]
          }
          event User Event {
            n133 = event-data() -> ("Module ID"=w62:i32)  [unwired: 1 in]
            n134 = call "Addressed to This Module.vi"("Module ID from Argument"=w62, "Module Admin"=w63) -> ("Addressed to this instance?"=w59:bool)  [unwired: 8 in, 1 out]
            n135 = case shown="True" w59 {
              tunnel: w61 -> [w65 w67]
              tunnel: [w65 refnum<visa-resource-name> refnum ("VISA resource name")] -> w60
              frame False {
              }
              frame True {
                n136 = call <instrlib>:"Close.vi"("VISA resource name"=w67) -> ()  [unwired: 10 in, 1 out]
              }
            }
          }
          event User Event {
            # "This module called the \"Local Instance.Start Continuous Acquisition\" local instance request."
            n137 = event-data() -> ("VISA resource name"=w69:refnum<visa-resource-name>)  [unwired: 1 in]
            n138 = call "Acquisition Polling Time--constant.vi"() -> ("Acquisition Polling Time (ms*"=w68:i32)  [unwired: 11 in]
          }
        }
        n139 = call "Connection Status Monitor.vi"("Module ID"=w33, "error in"=w39, "Acquisition Polling Time (ms* in"=w34, "VISA Refnum in"=w36) -> ("error out"=w35:errorcluster, "Acquisition Polling Time (ms* out"=w38:i32, "VISA Refnum out"=w37:refnum<visa-resource-name>)  [unwired: 5 in]
        n140 = call-dynamic "Delacor_lib_QMH_Error Handler - Helper Loop.vi"("Error Debug"=w42, "error in"=w35, "Message Queue in"=w43) -> ()  [unwired: 7 in, 2 out]
      }
      n141 = Unregister For Events(event registration refnum=w23) -> ()  [unwired: 1 in, 1 out]
    }
    frame Error {
      n142 = call "Synchronize Caller Events.vi"("Module Admin"=w301) -> ("Module Admin out"=w300:refnum<class "Delacor_lib_QMH_Cloneable Module Admin.lvclass">)  [unwired: 9 in, 1 out]
      n143 = property on="Property Node" class="Mod Admin"(reference=w300) -> ("Accessors:Module ID"=w299:i32)  [unwired: 1 in, 2 out]
      n144 = call-dynamic "Delacor_lib_QMH_Release Message Queue.vi"("error in"=w307, "Message Queue"=w298) -> ("error out"=w306:errorcluster)  [unwired: 9 in]
      n145 = call "Module Name--constant.vi"("Module ID"=w299) -> ("Module Name"=w304:string)  [unwired: 10 in]
      n146 = Format Into String(format string="An error occurred during initialization. %s is no longer running.", w304) -> (resulting string=w302:string)  [unwired: 2 in, 1 out]
      n147 = call "Error Reported.vi"("Additional Information"=w302, "Error"=w306, "Module ID"=w299) -> ()  [unwired: 8 in, 1 out]
    }
  }
  n148 = Merge Errors(w17, w16) -> (w18:errorcluster)
  n149 = call "Close Module.vi"("error in"=w18, "Wait for stop?"=w3, "Module Admin in"=w5) -> ("error out"=w14:errorcluster, "External Launch"=w2:bool, "Module Admin out"=w4:refnum<class "Delacor_lib_QMH_Cloneable Module Admin.lvclass">)  [unwired: 6 in]
  n150 = Unregister For Events(event registration refnum=w9, error in=w14) -> (error out=w13:errorcluster)
  "error out" <- w13
  n151 = case "External Launch?" shown="True" w2 {
    tunnel: w13 -> [_ w308]
    frame False {
    }
    frame True {
      n152 = case shown="No Error" w308 {
        frame No Error {
          n153 = invoke class="VI" method="FP.Close"() -> ()  [unwired: 3 in, 3 out]
        }
        frame Error {
          n154 = disable-structure shown="Default" {
            frame condition #0 (active) {
              n155 = invoke class="VI" method="FP.Open"("Activate"=TRUE ("Activate?")) -> ()  [unwired: 4 in, 5 out]
            }
            frame condition #1 {
              # "Don't show panel on error if running inside a built EXE."
            }
          }
        }
      }
    }
  }
  n156 = local write "Module Admin"(w4) -> ()
